vi "Support_Dialog.vi"(3 "message":string, 5 "error in (no error)":errorcluster) -> (19 "error out":errorcluster)   [LabVIEW 2009]
doc: "Dialog."
panel:
  out "message out":string
  in  "OK Button":bool
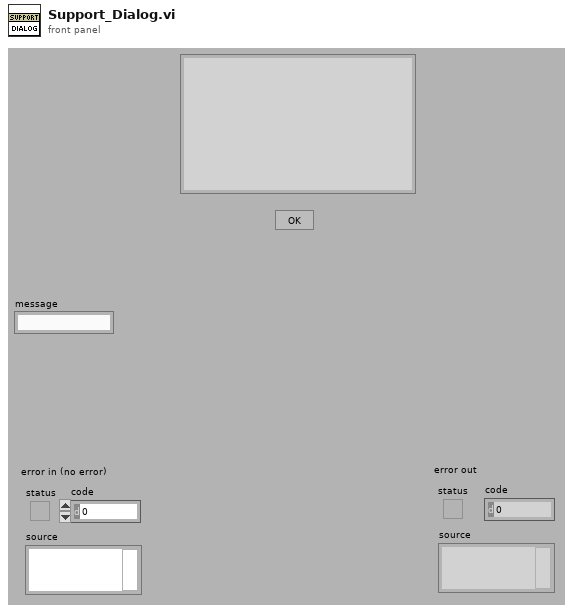
[diagram p1: front panel]
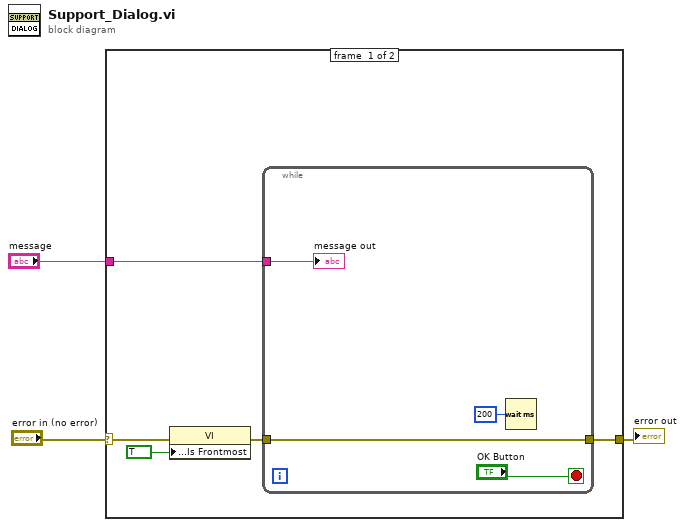
[diagram p0: block diagram]
diagram:
  n1 = case shown="No Error" "error in (no error)" {
    selector: "error in (no error)" -> [w7 w13]
    tunnel: "message" -> [w8 _]
    tunnel: [w5 w13] -> w1
    frame #0 {
      n2 = property class="VI"(error in=w7, "Front Panel Window:Is Frontmost"=TRUE) -> (error out=w6:errorcluster)  [unwired: 1 in, 1 out]
      n3 = while {
        tunnel: [w9] -> w5
        tunnel: w6 -> [w9]
        tunnel: w8 -> [w10]
        stop <- "OK Button" stop-if-true
        n4 = Wait (ms)(milliseconds to wait=u32 200) -> ()  [unwired: 1 out]
        "message out" <- w10
      }
    }
    frame #1 {
    }
  }
  "error out" <- w1
